vi "setAllDevices.vi"(8 "error in (no error)":errorcluster, 10 "deviceArray":refnum<class "device.lvclass">[](array[class]), 11 "DeviceArray.lvclass in":refnum<class "DeviceArray.lvclass">) -> (0 "error out":errorcluster, 3 "DeviceArray.lvclass out":refnum<class "DeviceArray.lvclass">)   [LabVIEW 2009, in "Tools.lvlib" / "DatabaseHelpers.lvlib" / "DeviceArray.lvclass"]
uses:
  DeviceArray.lvclass
  device/device.lvclass
  DeviceArray.lvclass/DeviceArray.ctl
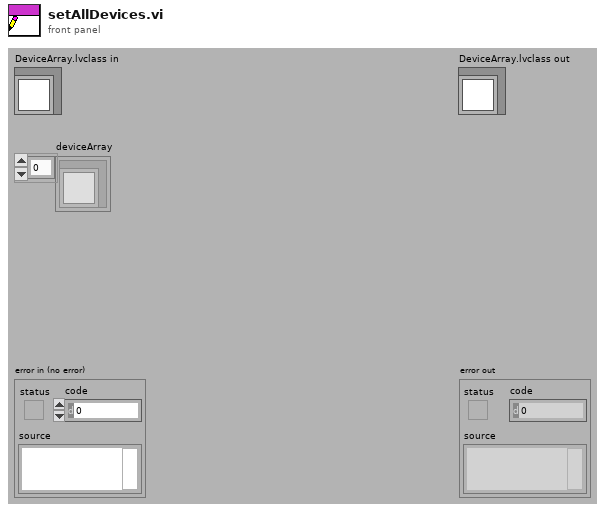
[diagram p1: front panel]
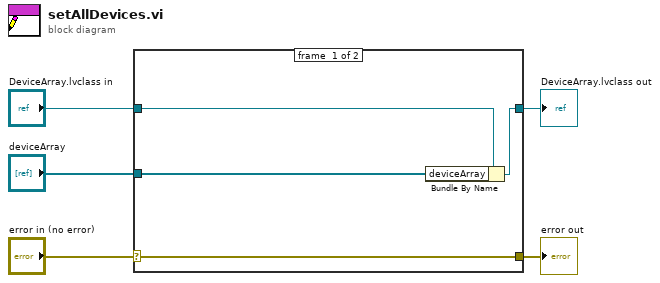
[diagram p0: block diagram]
diagram:
  n1 = case shown="No Error" "error in (no error)" {
    selector: "error in (no error)" -> [w9 w10]
    tunnel: [w9 w10] -> w4
    tunnel: [w7 w11] -> w2
    tunnel: "DeviceArray.lvclass in" -> [w8 w11]
    tunnel: "deviceArray" -> [w6 _]
    frame #0 {
      n2 = Bundle By Name(cluster=w8, "deviceArray"=w6) -> (w7:refnum<class "DeviceArray.lvclass">)
    }
    frame #1 {
    }
  }
  "error out" <- w4
  "DeviceArray.lvclass out" <- w2
